vi "Random Number#2.vi"(0 "Maximum":dbl=500.0, 1 "Minimum":dbl=100.0, 3 "error in (no error)":errorcluster) -> (6 "Integer":i64, 7 "Double":dbl, 8 "?":string, 9 "error out":errorcluster)   [LabVIEW 2020]
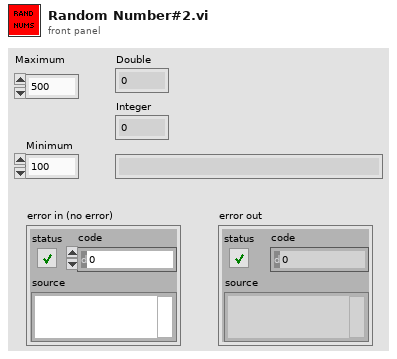
[diagram p1: front panel]
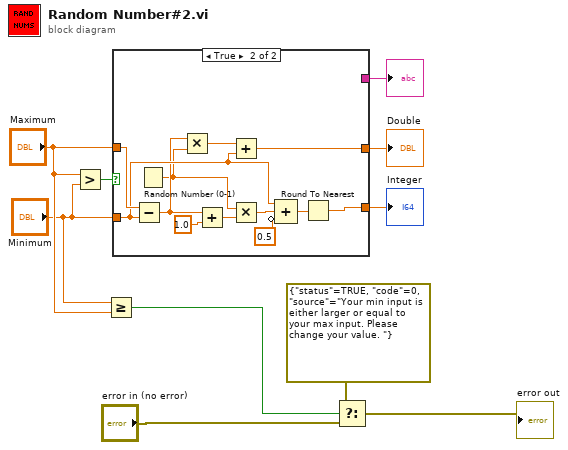
[diagram p0: block diagram]
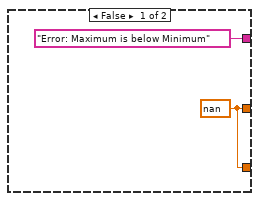
[diagram p2: hidden frame]
diagram:
  n1 = Greater?(x="Maximum", y="Minimum") -> (0:w10:bool)
  n2 = Greater Or Equal?(x="Minimum", y="Maximum") -> (x >= y?=w2:bool)
  n3 = case shown="True" w10 {
    tunnel: "Maximum" -> [_ w24]
    tunnel: "Minimum" -> [_ w18]
    tunnel: [w11 w22] -> w9
    tunnel: ["Error: Maximum is below Minimum" _] -> w8
    tunnel: [w11 w21] -> w7
    frame False {
      w11 = nan
    }
    frame True {
      n4 = Subtract(x=w24, y=w18) -> (x-y=w17:dbl)
      n5 = Random Number (0-1)() -> (number: 0 to 1=w15:dbl)
      n6 = Multiply(x=w17, y=w15) -> (x*y=w23:dbl)
      n7 = Add(x=w17, y=1.0) -> (x+y=w16:dbl)
      n8 = Add(x=w23, y=w18) -> (x+y=w22:dbl)
      n9 = Multiply(x=w15, y=w16) -> (x*y=w19:dbl)
      n10 = Compound Arithmetic op=ADD(w18, w19, invert 0.5 ("value")) -> (w20:dbl)
      n11 = Round To Nearest(number=w20) -> (nearest integer value=w21:dbl)
    }
  }
  "Double" <- w9
  "?" <- w8
  "Integer" <- w7
  n12 = Select(t=errorcluster {"status"=TRUE, "code"=0, "source"="Your min input is either larger or equal to your max input. Please change your value. "} ("error constant"), s=w2, f="error in (no error)") -> (s? t:f=→"error out":errorcluster)
